vi "Selected SS2 8-bit Frame Indices.vi"(1 "SS2 8-bit Frame Selection":T1) -> (0 "Selected 8-bit Frame Indices":i32[](array[numeric]))   [LabVIEW 2021, in "SwissSPAD.lvlib"]
uses:
  SwissSPAD.lvlib
  SwissSPAD 8-bit Frames Read.ctl
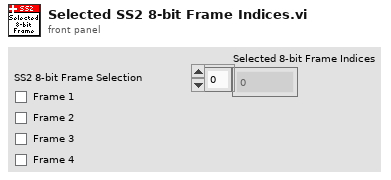
[diagram p1: front panel]
types:
  T1 = typedef "SwissSPAD.lvlib/SwissSPAD 8-bit Frames Read.ctl" = cluster{"Frame 1":bool, "Frame 2":bool, "Frame 3":bool, "Frame 4":bool}
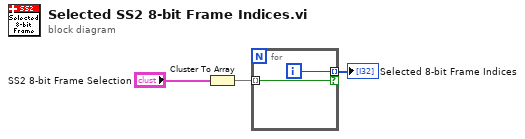
[diagram p0: block diagram]
diagram:
  n1 = Cluster To Array(cluster="SS2 8-bit Frame Selection") -> (array=w2:bool[])
  n2 = for {
    tunnel: w2 -> [w4] mode=indexing
    tunnel: [w5] -> w1 mode=indexing if=w4
    i -> [w5]
  }
  "Selected 8-bit Frame Indices" <- w1
